vi "Message Dequeue.vi"(6 "error in (no error)":errorcluster, 9 "Message Queue":refnum<queue>) -> (0 "error out":errorcluster, 1 "Value":variant, 2 "Message":string, 3 "Message Queue dup":refnum<queue>)   [LabVIEW 2013]
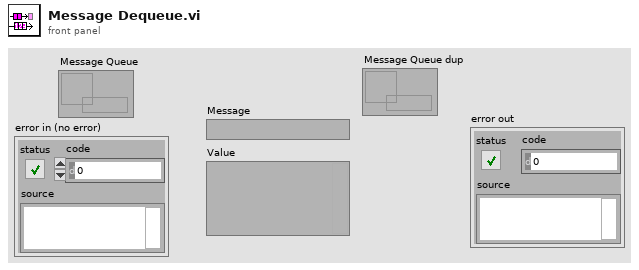
[diagram p1: front panel]
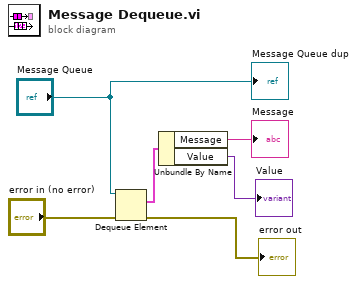
[diagram p0: block diagram]
diagram:
  n1 = Dequeue Element(queue="Message Queue", error in (no error)="error in (no error)") -> (element=w5:cluster{"Message":string, "Value":variant}, error out=→"error out":errorcluster)  [unwired: 1 in, 2 out]
  n2 = Unbundle By Name(w5) -> ("Message"=→"Message":string, "Value"=→"Value":variant)
  "Message Queue dup" <- "Message Queue"
